vi "Template Create Unique INI Filename.vi"(8 "error in (no error)":errorcluster) -> (0 "error out":errorcluster, 3 "INI Name":string)   [LabVIEW 2011]
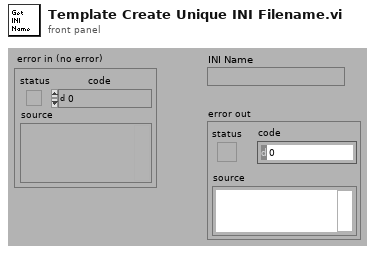
[diagram p1: front panel]
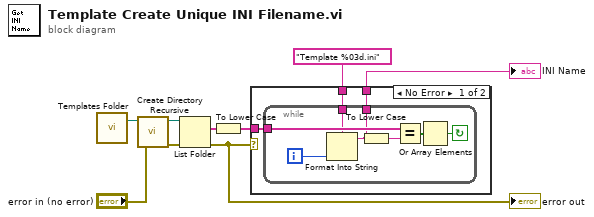
[diagram p0: block diagram]
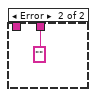
[diagram p2: hidden frame]
diagram:
  n1 = call "Templates Folder.vi"() -> ("Templates Folder"=w1:path)  [unwired: 1 in, 2 out]
  n2 = call <vilib>:"Create Directory Recursive.vi"("error in (no error)"="error in (no error)", "directory"=w1) -> ("error out"=w3:errorcluster, "directory copy"=w2:path)  [unwired: 1 in, 3 out]
  n3 = List Folder(path=w2, error in=w3) -> (filenames=w6:string[], error out=w9:errorcluster)  [unwired: 4 out]
  "error out" <- w9
  n4 = To Lower Case(string=w6) -> (all lower case string=w5:string[])
  n5 = case shown="No Error" w9 {
    tunnel: w5 -> [w12 _]
    tunnel: [w11 ""] -> w8
    tunnel: "Template %03d.ini" -> [w10 _]
    frame No Error {
      n6 = while {
        tunnel: [w15] -> w11
        tunnel: w12 -> [w19]
        tunnel: w10 -> [w16]
        i -> [w14]
        stop <- w17 continue-if-true
        n7 = Format Into String(format string=w16, w14) -> (resulting string=w15:string)  [unwired: 2 in, 1 out]
        n8 = To Lower Case(string=w15) -> (all lower case string=w13:string)
        n9 = Equal?(x=w19, y=w13) -> (x = y?=w18:bool[])
        n10 = Or Array Elements(Boolean array=w18) -> (logical OR=w17:bool)
      }
    }
    frame Error {
    }
  }
  "INI Name" <- w8
